vi "Cheby Pade fit_optimzation.vi"(0 "start":dbl=23.0 format="%.2f", 2 "number of points":u32=1000, 5 "end":dbl=41.5 format="%.2f", 7 "X-array":dbl[](array[numeric]), 9 "Y-array":dbl[](array[numeric])) -> ()   [LabVIEW 2025]
uses:
  <vilib>/gmath/NI_Gmath.lvlib
panel:
  out "Pade min SD":dbl=-0.0 format="%#_6e"
  out "best Pade m":i32
  out "best Pade p":i32
  out "best Pade Cheby n":u32
  out "XY Graph":cluster{dbl[], dbl[]}[](graph)
  out "best Cheby n":u32
  in  "Cheby only":bool
  out "Cheby min SD":dbl=99.0 format="%#_6e"
  out "Cheby n-countdown":i32=1
  out "p-countdown":i32=1
  out "m-countdown":i32=1
  in  "highest p-th derivative":i32=8
  in  "lowest p-th derivative":i32=2
  in  "highest Cheby order":u32=9
  in  "lowest Cheby order":u32=1
  in  "interpol-method":i32(ring)=1 items=["nearest", "linear", "spline", "cubic Hermite", "Lagrange"]
  # "1. Fitting procedures for a Cheby n-order (range is limited by controls lowest-Cheby order, highest Cheby-order)\n       For given Cheby n-order: perfrom Cheby only and Cheby-Pade approximation. \n       For given Cheby order: Pade p-order can be 1 to n but limited by the controls (lowest p-th derivative, highest p-th derivative)\n       For given Pade p-order, there are multiple (m, n) that satisfies p = m+n (m>=n).\n\n2. Find Cheby n-order from the Cheby-only fittings with minimum standard deviation (SD) \n\n3. Find (Cheby n-order, Pade-p, m. n) from Cheby-Pade fittings with mimimum SD."
  # "1. Note that the Chebyshev approximation is performed for normlaized x, i.e. [-1,1]. \nTherefore, x input for the Pade approximation  also requires the same normalization.\n2. Should be an ascending order"
  # "Constraints"
  # "Progress"
  # "Results"
  # "p=m+n\nm>=n\n\nIf P > Cheby order, the best Pade fitting is same with the result of Cheby-only fitting."
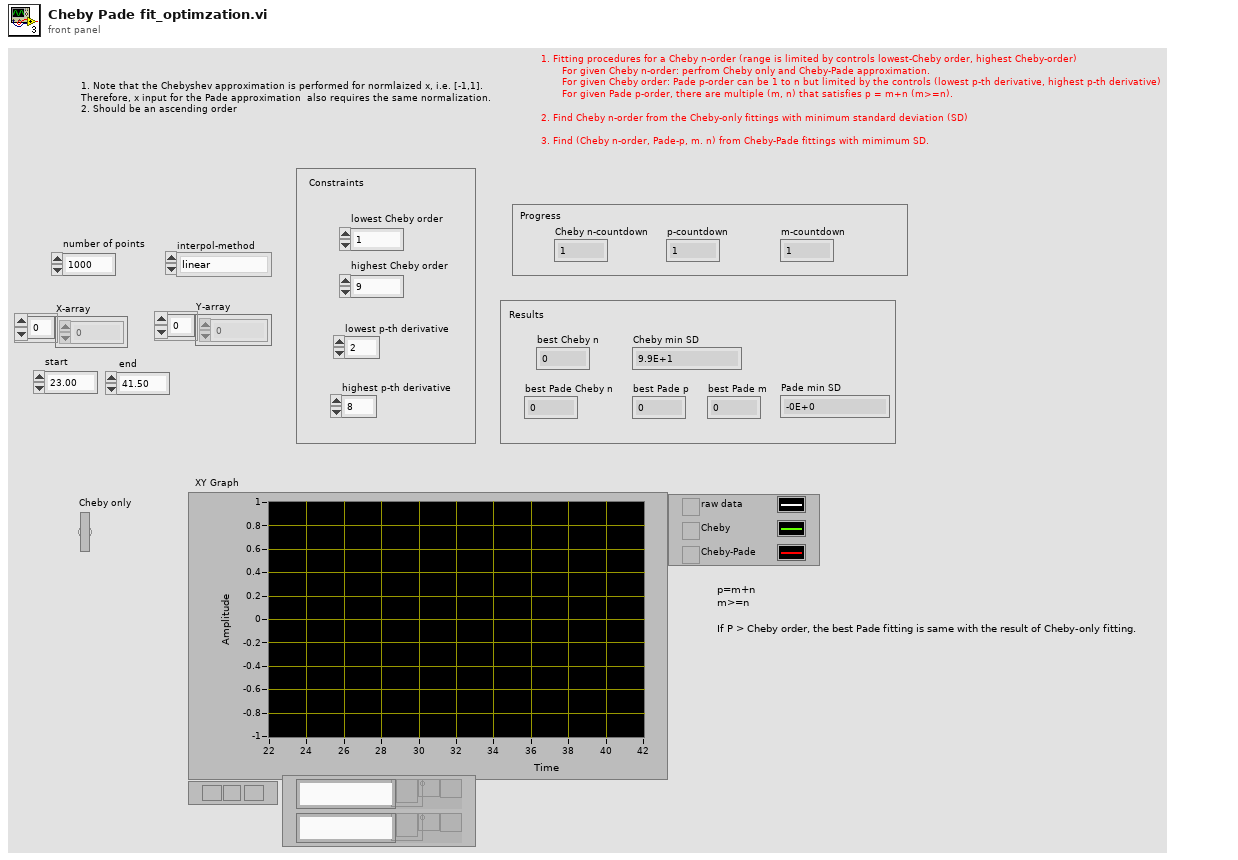
[diagram p1: front panel]
types:
  T1 = cluster{"raw data, Cheby, Pade":cluster{dbl[], "Pade_mn array":dbl[]}[], "x, Cheby residual, Cheby-Pade residual":dbl[], "Cheby SD":dbl, "Pade SD":dbl}
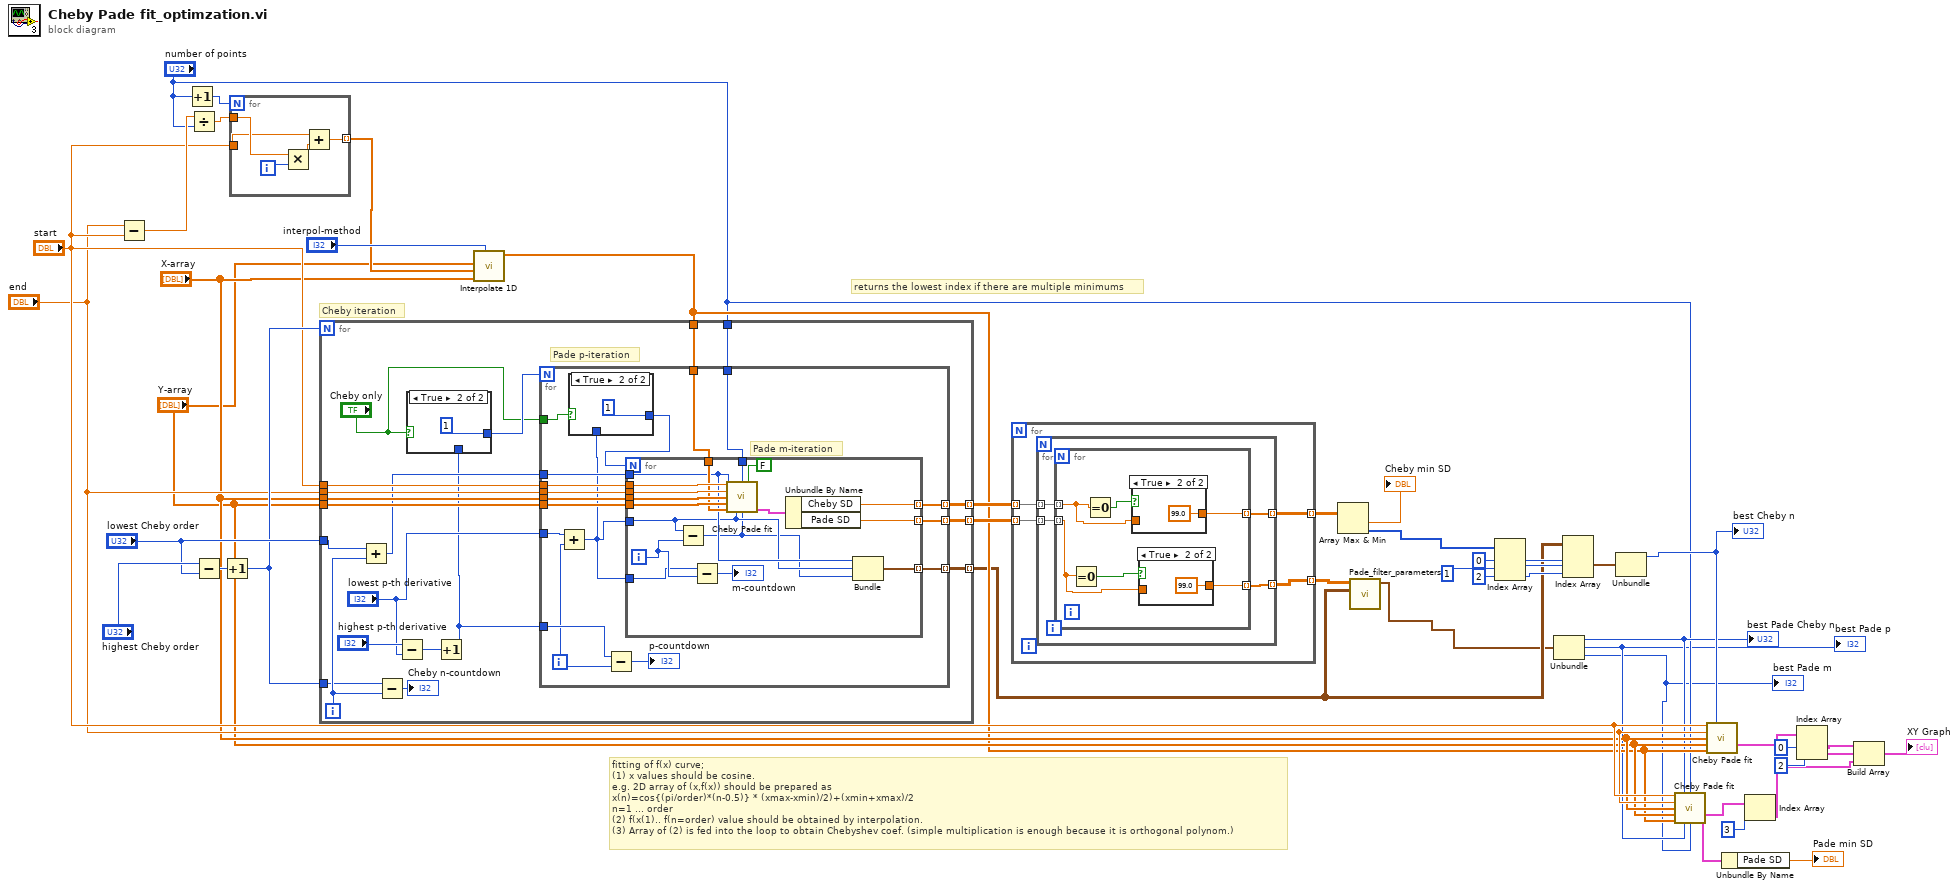
[diagram p0: block diagram]
diagram:
  # "returns the lowest index if there are multiple minimums"
  # "Cheby iteration"
  # "fitting of f(x) curve;\n(1) x values should be cosine.\ne.g. 2D array of (x,f(x)) should be prepared as \nx(n)=cos{(pi/order)*(n-0.5)} * (xmax-xmin)/2)+(xmin+xmax)/2 \nn=1 ... order\n(2) f(x(1).. f(n=order) value should be obtained by interpolation.\n(3) Array of (2) is fed into the loop to obtain Chebyshev coef. (simple multiplication is enough because it is orthogonal polynom.)"
  n1 = Subtract(x="end", y="start") -> (x-y=w45:dbl)
  n2 = Increment(x="number of points") -> (x+1=w43:u32)
  n3 = Divide(x=w45, y="number of points") -> (x/y=w44:dbl)
  n4 = Subtract(x="highest Cheby order", y="lowest Cheby order") -> (x-y=w39:u32)
  n5 = Increment(x=w39) -> (x+1=w37:u32)
  n6 = for {
    N: w43 -> [_]
    tunnel: "start" -> [w47]
    tunnel: w44 -> [w50]
    tunnel: [w46] -> w41 mode=indexing
    i -> [w49]
    n7 = Multiply(x=w50, y=w49) -> (x*y=w48:dbl)
    n8 = Add(x=w47, y=w48) -> (x+y=w46:dbl)
  }
  n9 = call <vilib>:"Interpolate 1D.vi"("method"="interpol-method", "xi"=w41, "X"="X-array", "Y"="Y-array") -> ("yi"=w10:dbl[])  [unwired: 5 in, 2 out]
  n10 = for {
    N: w37 -> [_]
    tunnel: "start" -> [w63]
    tunnel: "end" -> [w62]
    tunnel: "X-array" -> [w61]
    tunnel: "Y-array" -> [w60]
    tunnel: "lowest Cheby order" -> [w70]
    tunnel: "number of points" -> [w58]
    tunnel: w10 -> [w59]
    tunnel: w37 -> [w64]
    tunnel: [w56] -> w36 mode=indexing
    tunnel: [w55] -> w35 mode=indexing
    tunnel: [w54] -> w4 mode=indexing
    i -> [w65]
    # "Pade p-iteration"
    n11 = Add(x=w70, y=w65) -> (x+y=w57:u32)
    n12 = Subtract(x=w64, y=w65) -> (x-y=→"Cheby n-countdown":u32)
    n13 = Subtract(x="highest p-th derivative", y="lowest p-th derivative") -> (x-y=w69:i32)
    n14 = Increment(x=w69) -> (x+1=w52:i32)
    n15 = case shown="True" "Cheby only" {
      tunnel: [w71 1 ("x+1")] -> w53
      tunnel: w52 -> [w71 _]
      frame False {
      }
      frame True {
      }
    }
    n16 = for {
      N: w53 -> [_]
      tunnel: w63 -> [w89]
      tunnel: w62 -> [w88]
      tunnel: w61 -> [w87]
      tunnel: w60 -> [w86]
      tunnel: w57 -> [w85]
      tunnel: "lowest p-th derivative" -> [w84]
      tunnel: w58 -> [w83]
      tunnel: w59 -> [w82]
      tunnel: w52 -> [w80]
      tunnel: [w78] -> w56 mode=indexing
      tunnel: [w77] -> w55 mode=indexing
      tunnel: [w76] -> w54 mode=indexing
      tunnel: "Cheby only" -> [w75]
      i -> [w79]
      # "Pade m-iteration"
      n17 = Add(x=w84, y=w79) -> (x+y=w73:i32)
      n18 = case shown="True" w75 {
        tunnel: [w90 1 ("x+1")] -> w74
        tunnel: w73 -> [w90 _]
        frame False {
        }
        frame True {
        }
      }
      n19 = Subtract(x=w80, y=w79) -> (x-y=→"p-countdown":i32)
      n20 = for {
        N: w74 -> [_]
        tunnel: w89 -> [w108]
        tunnel: w88 -> [w107]
        tunnel: w87 -> [w106]
        tunnel: w86 -> [w105]
        tunnel: w85 -> [w95]
        tunnel: w73 -> [w94]
        tunnel: w83 -> [w102]
        tunnel: w82 -> [w101]
        tunnel: w73 -> [w99]
        tunnel: [w97] -> w78 mode=indexing
        tunnel: [w96] -> w77 mode=indexing
        tunnel: [w92] -> w76 mode=indexing
        i -> [w100]
        n21 = Subtract(x=w94, y=w100) -> (x-y=w93:i32)
        n22 = Subtract(x=w99, y=w100) -> (x-y=→"m-countdown":i32)
        n23 = call "Cheby Pade fit.vi"("start"=w108, "order"=w95, "number of points"=w102, "re-interpolate"=FALSE, "end"=w107, "X-array"=w106, "Y-array"=w105, "interpolated y"=w101, "p-the derivative"=w94, "m"=w93) -> ("fit results"=w104:T1)  [unwired: 5 out]
        n24 = Unbundle By Name(w104) -> ("Cheby SD"=w97:dbl, "Pade SD"=w96:dbl)
        n25 = Bundle(w95, w94, w93) -> (w92:cluster{u32, i32, i32})  [unwired: 1 in]
      }
    }
  }
  n26 = for {
    tunnel: [w112] -> w34 mode=indexing
    tunnel: [w111] -> w5 mode=indexing
    tunnel: w36 -> [w110] mode=indexing
    tunnel: w35 -> [w109] mode=indexing
    n27 = for {
      tunnel: [w116] -> w112 mode=indexing
      tunnel: [w115] -> w111 mode=indexing
      tunnel: w110 -> [w114] mode=indexing
      tunnel: w109 -> [w113] mode=indexing
      n28 = for {
        tunnel: [w121] -> w116 mode=indexing
        tunnel: [w119] -> w115 mode=indexing
        tunnel: w114 -> [w118] mode=indexing
        tunnel: w113 -> [w117] mode=indexing
        n29 = Equal To 0?(x=w117) -> (x = 0?=w120:bool)
        n30 = Equal To 0?(x=w118) -> (x = 0?=w122:bool)
        n31 = case shown="True" w122 {
          tunnel: [w125 99.0 ("Pade SD")] -> w121
          tunnel: w118 -> [w125 _]
          frame False {
          }
          frame True {
          }
        }
        n32 = case shown="True" w120 {
          tunnel: [w123 99.0 ("Pade SD")] -> w119
          tunnel: w117 -> [w123 _]
          frame False {
          }
          frame True {
          }
        }
      }
    }
  }
  n33 = Array Max & Min(array=w34) -> (min value=→"Cheby min SD":dbl, min index (indices)=w32:i32[])  [unwired: 2 out]
  n34 = call "Pade_filter_parameters.vi"("order cluster"=w4, "Array"=w5) -> ("Cluster"=w3:cluster{u32, i32, i32})  [unwired: 9 in]
  n35 = Index Array(array=w32, index #1=0 ("index"), index #2=1 ("index"), index #3=2 ("index")) -> (element #1=w28:i32, element #2=w27:i32, element #3=w26:i32)
  n36 = Unbundle(w3) -> (w9:u32, w7:i32, w6:i32)
  "best Pade Cheby n" <- w9
  "best Pade p" <- w7
  "best Pade m" <- w6
  n37 = Index Array(array=w4, index (dim 0)=w28, index (dim 1)=w27, index (dim 2)=w26) -> (element=w25:cluster{u32, i32, i32})
  n38 = Unbundle(w25) -> (w24:u32)  [unwired: 2 out]
  "best Cheby n" <- w24
  n39 = call "Cheby Pade fit.vi"("start"="start", "order"=w9, "number of points"="number of points", "end"="end", "X-array"="X-array", "Y-array"="Y-array", "interpolated y"=w10, "p-the derivative"=w7, "m"=w6) -> ("XY Graph"=w17:cluster{dbl[], dbl[]}[], "fit results"=w2:T1)  [unwired: 1 in, 4 out]
  n40 = call "Cheby Pade fit.vi"("start"="start", "order"=w24, "end"="end", "X-array"="X-array", "Y-array"="Y-array", "interpolated y"=w10) -> ("XY Graph"=w23:cluster{dbl[], dbl[]}[])  [unwired: 4 in, 5 out]
  n41 = Unbundle By Name(w2) -> ("Pade SD"=→"Pade min SD":dbl)
  n42 = Index Array(array=w17, index=3) -> (element=w15:cluster{dbl[], dbl[]})
  n43 = Index Array(array=w23, index #1=0 ("index"), index #2=2 ("index")) -> (element #1=w20:cluster{dbl[], dbl[]}, element #2=w19:cluster{dbl[], dbl[]})
  n44 = Build Array(w20, w19, w15) -> (→"XY Graph":cluster{dbl[], dbl[]}[])
